vi "FA.vi"(8 "数组大小":i32, 9 "Mode":bool, 10 "buf":u8[](array[numeric]) format="%02x") -> ()   [LabVIEW 2015]
doc: "Mode = 1? RTU；ASCII;"
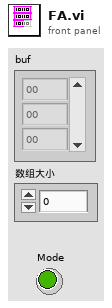
[diagram p1: front panel]
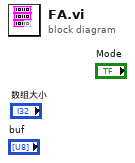
[diagram p0: block diagram]
diagram:
